vi "Corr Transducers Reload All.vi"(8 "error in":errorcluster, 11 "transducers in":cluster{"channels":T1[], "last path":path} {"channels"."Phase index" min=1 step=1}) -> (0 "error out":errorcluster, 3 "transducers out":cluster{"channels":T1[], "last path":path} {"channels"."Phase index" min=1 step=1})   [LabVIEW 2018]
doc: "Reloads all transducers in the list. If no path is available it will replace the transducer with empty record. It will generate error if some tranducer is not loaded sucessfully."
uses:
  Corr Tranducer Item.ctl
  octave/infolib.lvlibp/Private/Get key polymorph parts/GetString.vi
  <vilib>/Utility/error.llb/Error Cluster From Error Code.vi
  <vilib>/ErrorRing/Error Ring.xnode
  <vilib>/regexp/Match Regular Expression.xnode
  octave/infolib.lvlibp
panel:
  # "ADC:"
  # "ADC:"
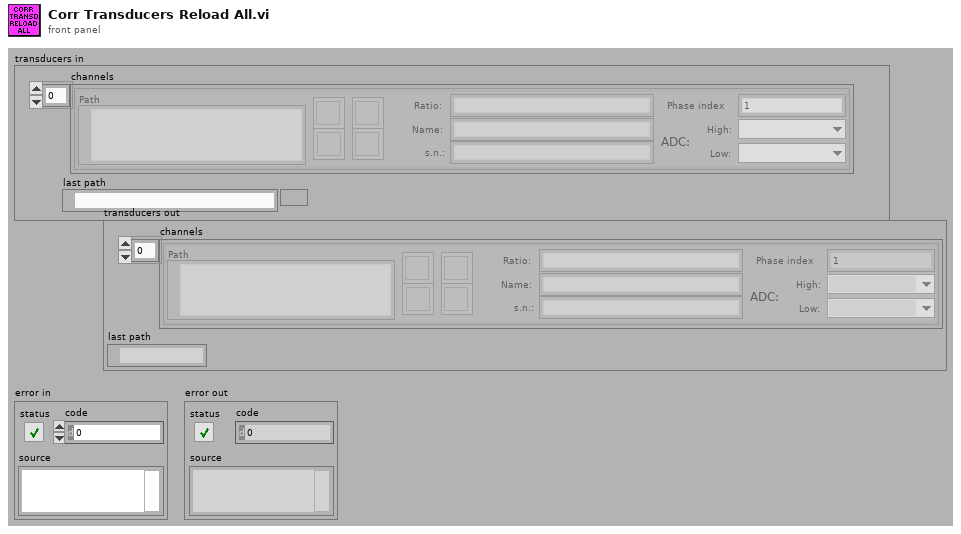
[diagram p1: front panel]
types:
  T1 = typedef "Corr Tranducer Item.ctl" = cluster{"Path":path, "Ratio:":string, "Name:":string, "btn rem":bool, "btn up":bool, "btn down":bool, "s.n.:":string, "btn open":bool, "ratio o/i":dbl, "chn hi":u16, "chn lo":u16, "Phase index":i32}
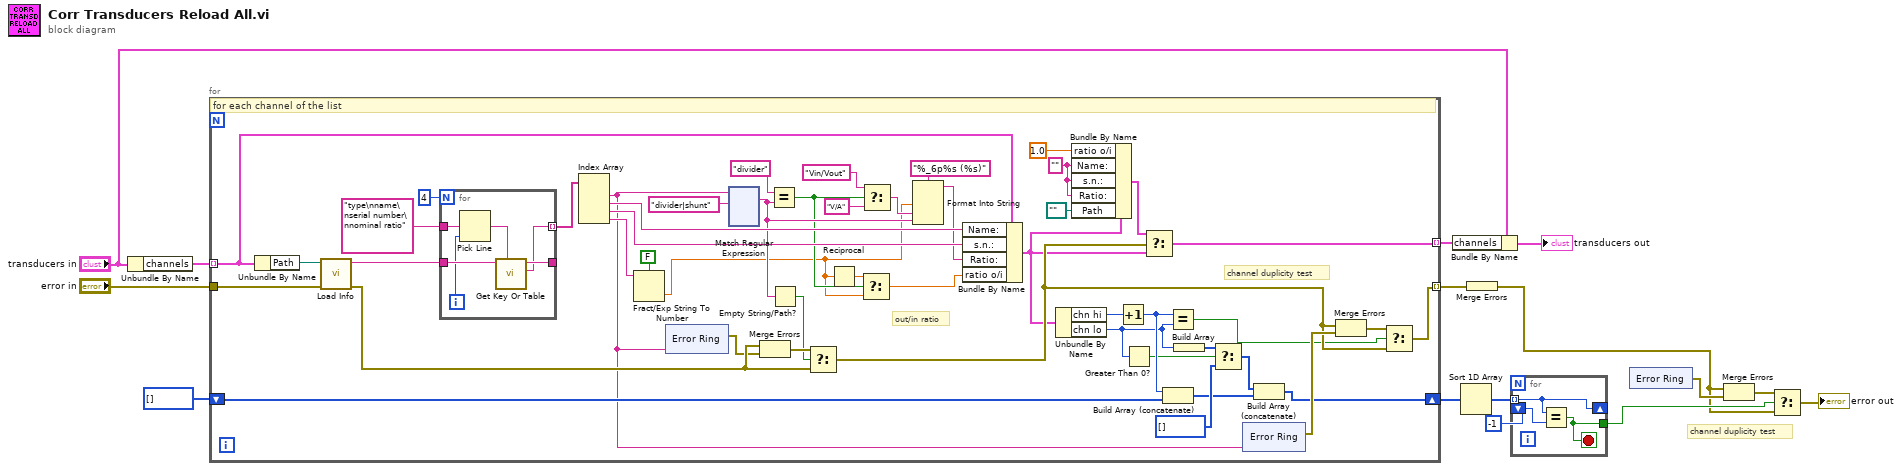
[diagram p0: block diagram]
diagram:
  # "channel duplicity test"
  n1 = Unbundle By Name("transducers in") -> ("channels"=w15:T1[])
  n2 = for {
    tunnel: w15 -> [w53] mode=indexing
    tunnel: [w38] -> w12 mode=indexing
    tunnel: "error in" -> [w63]
    tunnel: [w23] -> w11 mode=indexing
    shift-right: [w22] -> w8
    shift-left: i32[] [] -> [w36]
    w16 = "" ("Name:")
    # "channel duplicity test"
    # "out/in ratio"
    # "for each channel of the list"
    n3 = Unbundle By Name(w53) -> ("Path"=w64:path)
    n4 = call "Load Info.vi"("error in"=w63, "filename"=w64) -> ("error out"=w56:errorcluster, "info data"=w61:string)  [unwired: 8 in]
    n5 = for {
      N: 4 -> [_]
      tunnel: "type\nname\nserial number\nnominal ratio" ("key description") -> [w197]
      tunnel: w61 -> [w196]
      tunnel: [w195] -> _
      tunnel: [w194] -> w60 mode=indexing
      i -> [w193]
      n6 = Pick Line(multi-line string=w197, line index=w193) -> (output string=w198:string)  [unwired: 1 in]
      n7 = call-poly "Get Key Or Table.vi"("key description"=w198, "info data"=w196) -> ("value"=w194:string, "info data out"=w195:string)  [unwired: 6 in, 2 out]
    }
    n8 = Index Array(array=w60) -> (element #1=w21:string, element #2=w52:string, element #3=w51:string, element #4=w50:string)  [unwired: 4 in]
    n9 = Fract/Exp String To Number(use system decimal point (T)=FALSE, string=w50) -> (number=w40:dbl)  [unwired: 2 in, 1 out]
    n10 = xnode "Error Ring"("parameter 0"=w21) -> ("error out"=w55:errorcluster)
    n11 = xnode "Match Regular Expression"("input string"=w21, "regular expression"="divider|shunt") -> ("whole match"=w44:string)  [unwired: 4 in, 4 out]
    n12 = Merge Errors(w56, w55) -> (w57:errorcluster)
    n13 = Equal?(x="divider", y=w44) -> (x = y?=w42:bool)
    n14 = Empty String/Path?(string/path=w44) -> (empty?=w54:bool)
    n15 = Select(t=w57, s=w54, f=w56) -> (s? t:f=w25:errorcluster)
    n16 = Reciprocal(x=w40) -> (1/x=w41:dbl)
    n17 = Select(t=w41, s=w42, f=w40) -> (s? t:f=w39:dbl)
    n18 = Select(t="Vin/Vout" ("x"), s=w42, f="V/A") -> (s? t:f=w45:string)
    n19 = Format Into String(format string="%_6p%s (%s)", w40, w45, w44) -> (resulting string=w43:string)  [unwired: 2 in, 1 out]
    n20 = Bundle By Name(cluster=w53, "Name:"=w52, "s.n.:"=w51, "Ratio:"=w43, "ratio o/i"=w39) -> (w20:T1)
    n21 = Unbundle By Name(w20) -> ("chn hi"=w35:u16, "chn lo"=w32:u16)
    n22 = Bundle By Name(cluster=w20, "ratio o/i"=1.0, "Name:"=w16, "s.n.:"=w16, "Ratio:"=w16, "Path"=path "") -> (w19:T1)
    n23 = Increment(x=w35) -> (x+1=w34:u16)
    n24 = Greater Than 0?(x=w32) -> (x > 0?=w33:bool)
    n25 = Select(t=w19, s=w25, f=w20) -> (s? t:f=w38:T1)
    n26 = Build Array (concatenate)(w34, w36) -> (w29:i32[])
    n27 = Equal?(x=w34, y=w32) -> (x = y?=w24:bool)
    n28 = Build Array(w32) -> (w31:u16[])
    n29 = Select(t=w31, s=w33, f=i32[] []) -> (s? t:f=w28:i32[])
    n30 = xnode "Error Ring"("parameter 0"=w21) -> ("error out"=w27:errorcluster)
    n31 = Build Array (concatenate)(w28, w29) -> (w22:i32[])
    n32 = Merge Errors(w25, w27) -> (w26:errorcluster)
    n33 = Select(t=w26, s=w24, f=w25) -> (s? t:f=w23:errorcluster)
  }
  n34 = Bundle By Name(cluster="transducers in", "channels"=w12) -> (→"transducers out":cluster{"channels":T1[], "last path":path})
  n35 = Sort 1D Array(array=w8) -> (sorted array=w7:i32[])
  n36 = Merge Errors(w11) -> (w2:errorcluster)
  n37 = for {
    tunnel: w7 -> [w201] mode=indexing
    shift-right: [w201] -> _
    shift-left: -1 -> [w200]
    tunnel: [w199] -> w3
    stop <- w199 stop-if-true
    n38 = Equal?(x=w201, y=w200) -> (x = y?=w199:bool)
  }
  n39 = xnode "Error Ring"() -> ("error out"=w4:errorcluster)
  n40 = Merge Errors(w2, w4) -> (w5:errorcluster)
  n41 = Select(t=w5, s=w3, f=w2) -> (s? t:f=→"error out":errorcluster)
